vi "DAQ.Create DAQmx Async Read.vi"(8 "error in (no error)":errorcluster, 11 "Array":refnum<k21>[](array[refnum])) -> (0 "error out":errorcluster, 3 "VI out":refnum<vi>)   [LabVIEW 2019, in "DAQmx.lvclass"]
uses:
  DAQmx.lvclass
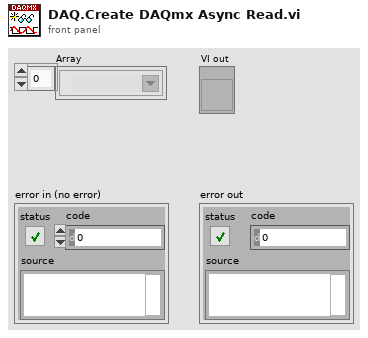
[diagram p1: front panel]
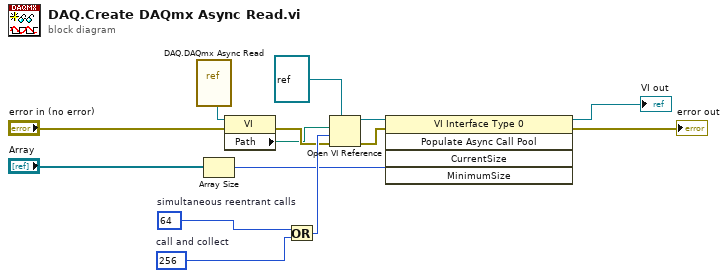
[diagram p0: block diagram]
diagram:
  w8 = 64  # simultaneous reentrant calls
  w10 = 256  # call and collect
  n1 = vi-ref "DAQ.DAQmx Async Read.vi"() -> (w6:refnum<vi>)
  n2 = Array Size(array="Array") -> (size(s)=w7:i32)
  n3 = property class="VI"(reference=w6, error in="error in (no error)") -> (error out=w2:errorcluster, "Path"=w1:path)  [unwired: 1 out]
  n4 = Or(x=w8, y=w10) -> (x .or. y?=w9:i32)
  n5 = Open VI Reference(type specifier VI Refnum (for type only)=refnum<vi> refnum, vi path=w1, options=w9, error in (no error)=w2) -> (vi reference=w4:refnum<vi>, error out=w5:errorcluster)  [unwired: 2 in]
  n6 = invoke class="VI Interface Type 0" method="Populate Async Call Pool"(reference=w4, error in=w5, "MinimumSize"=w7) -> (reference out=→"VI out":refnum<vi>, error out=→"error out":errorcluster)  [unwired: 2 in, 3 out]
